vi "ASDA-A2.vi"(5 "Dec":i32, 6 "Address":u16(ring) items=["1", "2"], 7 "Acc":i32, 8 "Torque\\Speed":i32, 9 "Mode":T1(ring)=enum."Set Speed", 10 "VISA resource name":refnum<visa-resource-name>="COM1") -> (1 "Speed":i32, 2 "Error":bool)   [LabVIEW 2024]
panel:
  out "substring":string
  out "crc check result":string
  out "Tact Time":u32
  out "send string":string
  out "Numeric":u8 format="%.0x"
  out "read string":string
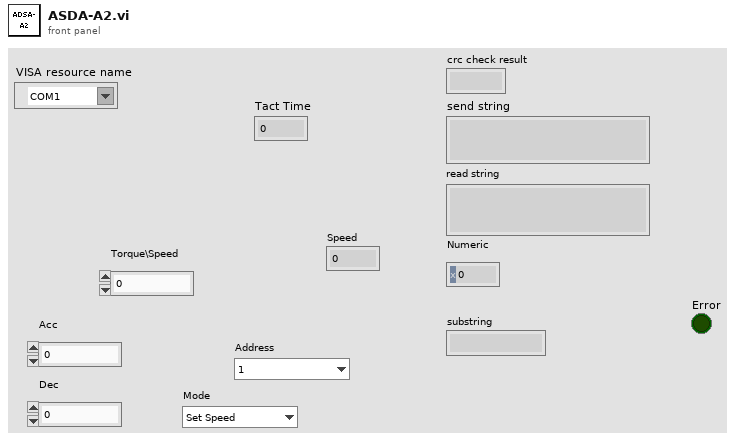
[diagram p1: front panel]
types:
  T1 = enum16{"Set Torque", "Set Speed", "Read Speed", "Set Acc/Dec"}
  T2 = cluster{"VISA resource name":refnum<visa-resource-name>, "baud rate":u32, "data bits":u16, "parity":u16, "stop bits":u16, "flow control":u16, "Read TimeOut (ms)":u32, "Byte Read Count(999Exit)":u32, "Read End Str":bool, "End String":string}
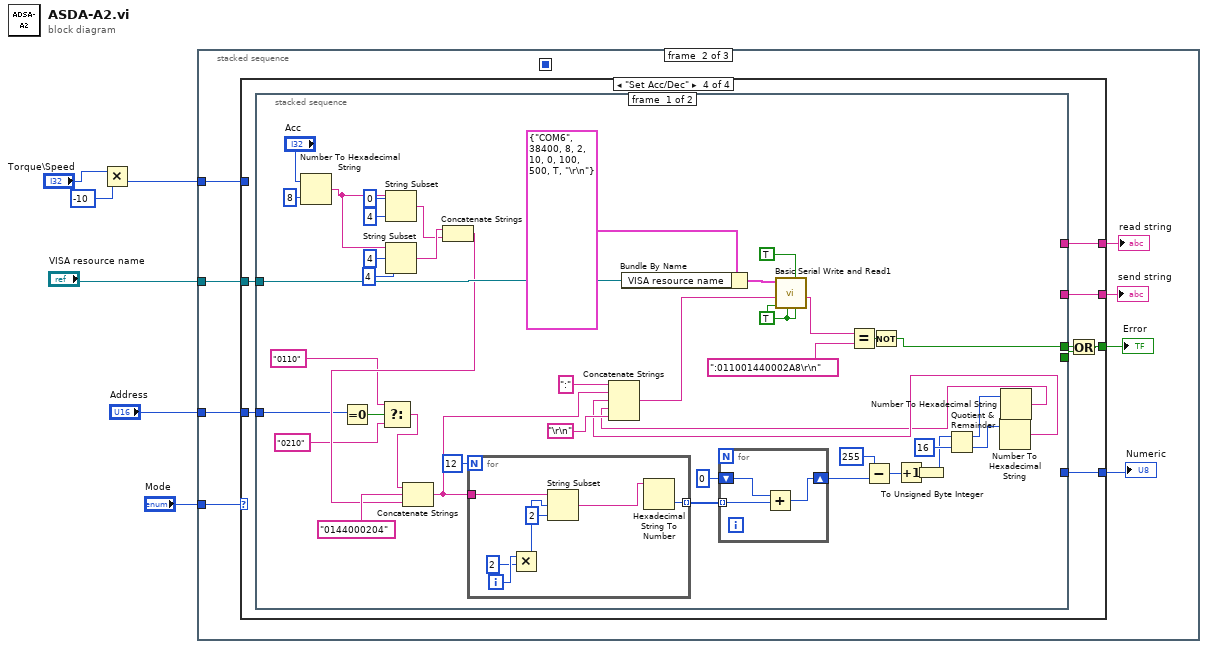
[diagram p0: block diagram]
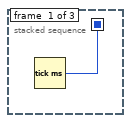
[diagram p2: hidden frame]
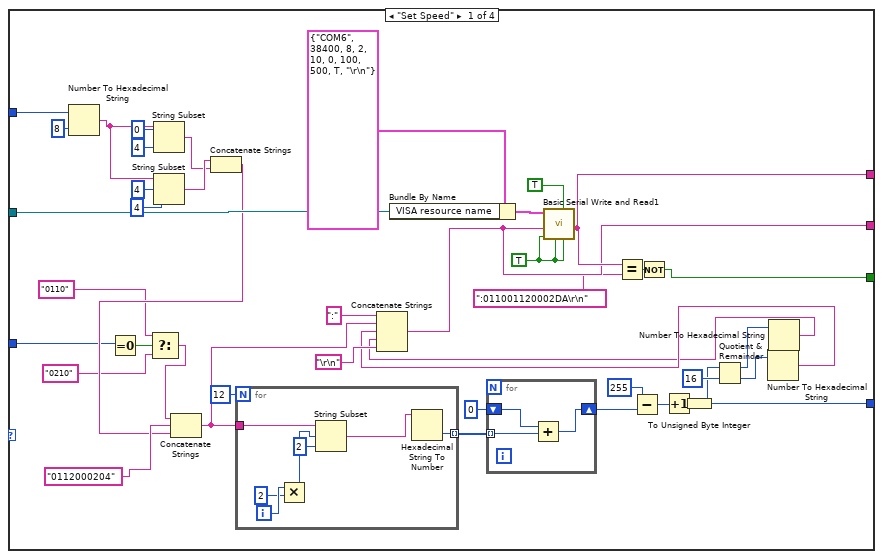
[diagram p3: hidden frame]
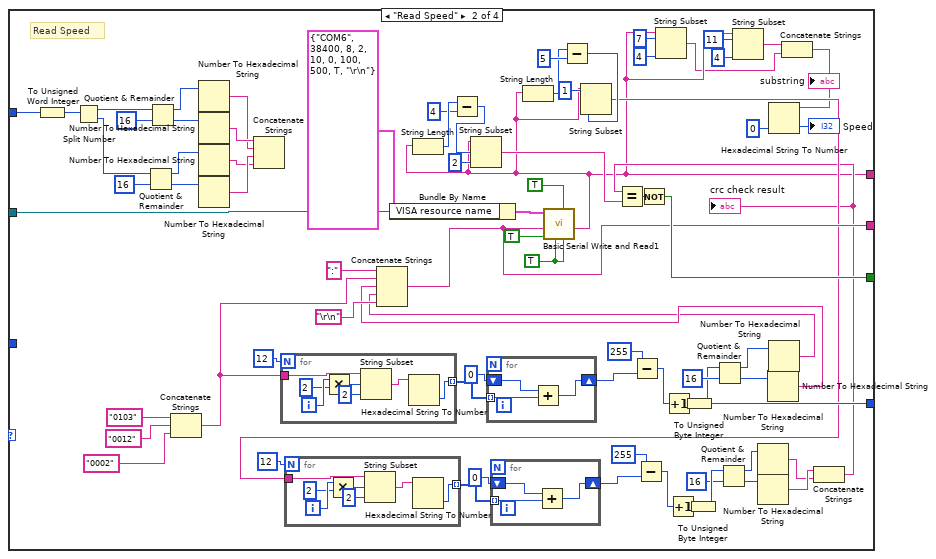
[diagram p4: hidden frame]
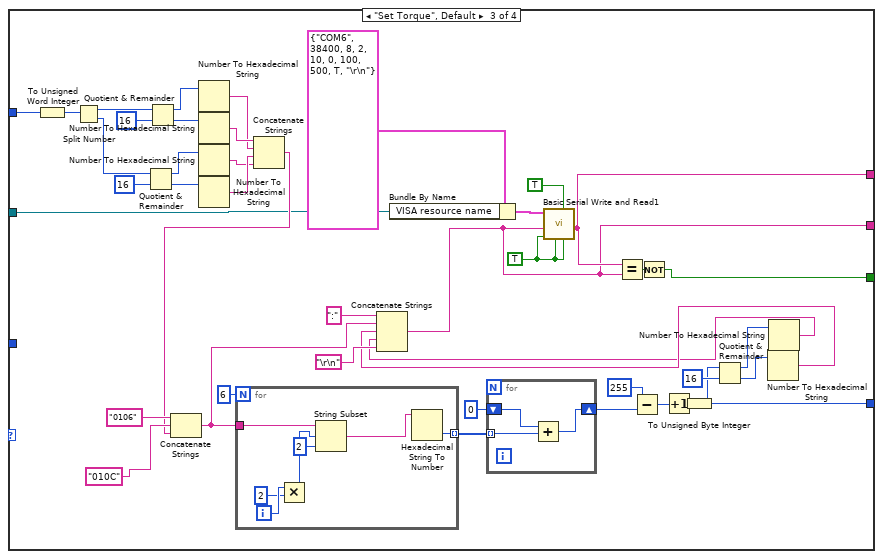
[diagram p5: hidden frame]
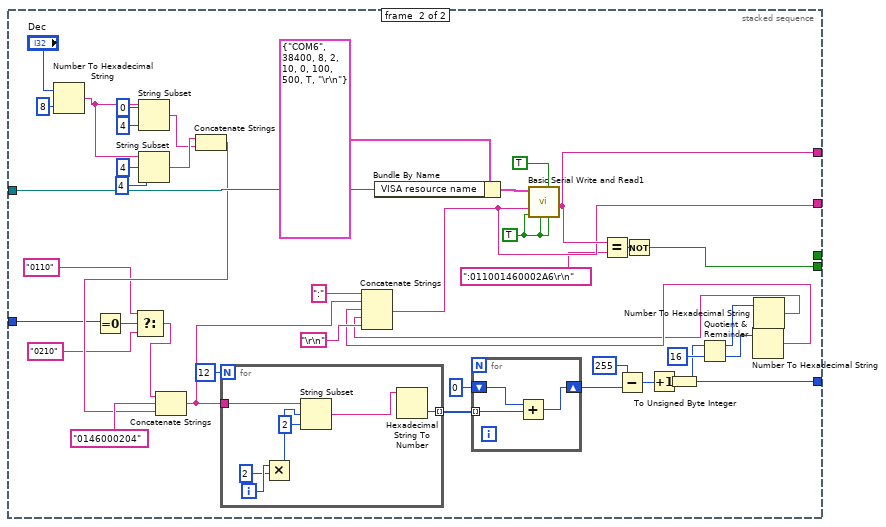
[diagram p6: hidden frame]
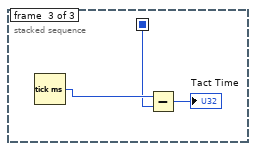
[diagram p7: hidden frame]
diagram:
  n1 = Multiply(x="Torque\\Speed", y=-10) -> (x*y=w3:i32)
  n2 = stacked-sequence {
    seq-local: [w7 _ _] -> [_ _ w329]
    tunnel: w3 -> [_ w15 _]
    tunnel: "VISA resource name" -> [_ w14 _]
    tunnel: "Mode" -> [_ w13 _]
    tunnel: "Address" -> [_ w8 _]
    frame #0 {
      n3 = Tick Count (ms)() -> (millisecond timer value=w7:u32)
    }
    frame #1 {
      n4 = case shown="\"Set Acc/Dec\"" w13 {
        tunnel: w15 -> [w32 w126 w187 _]
        tunnel: w14 -> [w38 w110 w170 w223]
        tunnel: [w36 w108 w168 w222] -> w12
        tunnel: [w35 w107 w167 w218] -> w11
        tunnel: [w34 w73 w166 w221] -> w10
        tunnel: [w33 w106 w165 w220] -> w9
        tunnel: w8 -> [w17 _ _ w219]
        frame "Set Speed" {
          w16 = TRUE ("read")
          n5 = Number To Hexadecimal String(1:i16 8 ("width (-)"), 2:w32) -> (0:w29:string)
          n6 = Equal To 0?(x=w17) -> (x = 0?=w22:bool)
          n7 = Select(t="0110" ("string to write"), s=w22, f="0210" ("string to write")) -> (s? t:f=w20:string)
          n8 = String Subset(string=w29, offset (0)=0, length (rest)=4 ("length (rest)")) -> (substring=w24:string)
          n9 = String Subset(string=w29, offset (0)=4, length (rest)=4 ("length (rest)")) -> (substring=w25:string)
          n10 = Concatenate Strings(w25, w24) -> (w23:string)
          n11 = Concatenate Strings(w20, "0112000204" ("string to write"), w23) -> (w44:string)
          n12 = for {
            N: 12 -> [_]
            tunnel: w44 -> [w64]
            tunnel: [w58] -> w52 mode=indexing
            i -> [w62]
            n13 = Multiply(x=w62, y=2) -> (x*y=w60:i32)
            n14 = String Subset(string=w64, offset (0)=w60, length (rest)=2 ("length (rest)")) -> (substring=w59:string)
            n15 = Hexadecimal String To Number(string=w59) -> (number=w58:u32)  [unwired: 2 in, 1 out]
          }
          n16 = Bundle By Name(cluster=T2 {"VISA resource name"="COM6", "baud rate"=38400, "data bits"=8, "parity"=2, "stop bits"=10, "flow control"=0, "Read TimeOut (ms)"=100, "Byte Read Count(999Exit)"=500, "Read End Str"=TRUE, "End String"="\r\n"} ("Setting"), "VISA resource name"=w38) -> (w39:T2)
          n17 = for {
            shift-right: [w65] -> w49
            shift-left: u32 0 -> [w67]
            tunnel: w52 -> [w66] mode=indexing
            n18 = Add(x=w67, y=w66) -> (x+y=w65:u32)
          }
          n19 = Subtract(x=u32 255, y=w49) -> (x-y=w50:u32)
          n20 = Increment(x=w50) -> (x+1=w48:u32)
          n21 = To Unsigned Byte Integer(number=w48) -> (unsigned 8bit integer=w36:u8)
          n22 = Quotient & Remainder(x=w36, y=u32 16) -> (x-y*floor(x/y)=w46:u32, floor(x/y)=w45:u32)
          n23 = Number To Hexadecimal String(2:w45) -> (0:w42:string)  [unwired: 1 in]
          n24 = Number To Hexadecimal String(2:w46) -> (0:w41:string)  [unwired: 1 in]
          n25 = Concatenate Strings(":" ("string to write"), w44, w42, w41, "\r\n") -> (w33:string)
          n26 = call "Basic Serial Write and Read1.vi"("read"=w16, "write"=TRUE, "Close"=w16, "Open"=w16, "string to write"=w33, "Setting"=w39) -> ("read string"=w34:string)  [unwired: 3 in, 2 out]
          n27 = Equal?(x=w34, y=":011001120002DA\r\n") -> (x = y?=w37:bool)
          n28 = Not(x=w37) -> (.not. x?=w35:bool)
        }
        frame "Read Speed" {
          w68 = TRUE ("read")
          # "Read Speed"
          n29 = To Unsigned Word Integer(number=w126) -> (unsigned 16bit integer=w125:u16)
          n30 = Split Number(x=w125) -> (hi(x)=w122:u8, lo(x)=w117:u8)
          n31 = Quotient & Remainder(x=w117, y=u8 16) -> (x-y*floor(x/y)=w119:u8, floor(x/y)=w118:u8)
          n32 = Quotient & Remainder(x=w122, y=u8 16) -> (x-y*floor(x/y)=w123:u8, floor(x/y)=w124:u8)
          n33 = Concatenate Strings("0103" ("string to write"), "0012" ("string"), "0002" ("string")) -> (w130:string)
          n34 = Number To Hexadecimal String(2:w123) -> (0:w115:string)  [unwired: 1 in]
          n35 = Number To Hexadecimal String(2:w124) -> (0:w116:string)  [unwired: 1 in]
          n36 = Number To Hexadecimal String(2:w119) -> (0:w113:string)  [unwired: 1 in]
          n37 = Number To Hexadecimal String(2:w118) -> (0:w114:string)  [unwired: 1 in]
          n38 = Concatenate Strings(w116, w115, w114, w113) -> ()  [unwired: 1 out]
          n39 = for {
            N: 12 -> [_]
            tunnel: w130 -> [w160]
            tunnel: [w154] -> w138 mode=indexing
            i -> [w158]
            n40 = Multiply(x=w158, y=2) -> (x*y=w156:i32)
            n41 = String Subset(string=w160, offset (0)=w156, length (rest)=2 ("length (rest)")) -> (substring=w155:string)
            n42 = Hexadecimal String To Number(string=w155) -> (number=w154:u32)  [unwired: 2 in, 1 out]
          }
          n43 = Bundle By Name(cluster=T2 {"VISA resource name"="COM6", "baud rate"=38400, "data bits"=8, "parity"=2, "stop bits"=10, "flow control"=0, "Read TimeOut (ms)"=100, "Byte Read Count(999Exit)"=500, "Read End Str"=TRUE, "End String"="\r\n"} ("Setting"), "VISA resource name"=w110) -> (w111:T2)
          n44 = for {
            shift-right: [w161] -> w135
            shift-left: u32 0 -> [w163]
            tunnel: w138 -> [w162] mode=indexing
            n45 = Add(x=w163, y=w162) -> (x+y=w161:u32)
          }
          n46 = Subtract(x=u32 255, y=w135) -> (x-y=w136:u32)
          n47 = Increment(x=w136) -> (x+1=w134:u32)
          n48 = To Unsigned Byte Integer(number=w134) -> (unsigned 8bit integer=w108:u8)
          n49 = Quotient & Remainder(x=w108, y=u32 16) -> (x-y*floor(x/y)=w132:u32, floor(x/y)=w131:u32)
          n50 = Number To Hexadecimal String(2:w131) -> (0:w128:string)  [unwired: 1 in]
          n51 = Number To Hexadecimal String(2:w132) -> (0:w127:string)  [unwired: 1 in]
          n52 = Concatenate Strings(":" ("string to write"), w130, w128, w127, "\r\n") -> (w106:string)
          n53 = call "Basic Serial Write and Read1.vi"("read"=w68, "write"=TRUE, "Close"=w68, "Open"=TRUE, "string to write"=w106, "Setting"=w111) -> ("read string"=w73:string)  [unwired: 3 in, 2 out]
          n54 = String Length(string=w73) -> (length=w102:i32)
          n55 = Subtract(x=w102, y=4) -> (x-y=w100:i32)
          n56 = String Subset(string=w73, offset (0)=w100, length (rest)=2 ("length (rest)")) -> (substring=w81:string)
          n57 = String Length(string=w73) -> (length=w97:i32)
          n58 = Subtract(x=w97, y=5) -> (x-y=w95:i32)
          n59 = String Subset(string=w73, offset (0)=1, length (rest)=w95) -> (substring=w83:string)
          n60 = for {
            N: 12 -> [_]
            tunnel: w83 -> [w150]
            tunnel: [w144] -> w86 mode=indexing
            i -> [w148]
            n61 = Multiply(x=w148, y=2) -> (x*y=w146:i32)
            n62 = String Subset(string=w150, offset (0)=w146, length (rest)=2 ("length (rest)")) -> (substring=w145:string)
            n63 = Hexadecimal String To Number(string=w145) -> (number=w144:u32)  [unwired: 2 in, 1 out]
          }
          n64 = for {
            shift-right: [w151] -> w89
            shift-left: u32 0 -> [w153]
            tunnel: w86 -> [w152] mode=indexing
            n65 = Add(x=w153, y=w152) -> (x+y=w151:u32)
          }
          n66 = Subtract(x=u32 255, y=w89) -> (x-y=w88:u32)
          n67 = String Subset(string=w73, offset (0)=7, length (rest)=4 ("length (rest)")) -> (substring=w71:string)
          n68 = Increment(x=w88) -> (x+1=w90:u32)
          n69 = To Unsigned Byte Integer(number=w90) -> (unsigned 8bit integer=w94:u8)
          n70 = Quotient & Remainder(x=w94, y=u32 16) -> (x-y*floor(x/y)=w92:u32, floor(x/y)=w93:u32)
          n71 = String Subset(string=w73, offset (0)=11, length (rest)=4 ("length (rest)")) -> (substring=w72:string)
          n72 = Number To Hexadecimal String(2:w92) -> (0:w79:string)  [unwired: 1 in]
          n73 = Number To Hexadecimal String(2:w93) -> (0:w80:string)  [unwired: 1 in]
          n74 = Concatenate Strings(w72, w71) -> (w70:string)
          "substring" <- w70
          n75 = Hexadecimal String To Number(string=w70, default (0uL)=0 ("default (0 U32)")) -> (number=→"Speed":i32)  [unwired: 1 in, 1 out]
          n76 = Concatenate Strings(w80, w79) -> (w82:string)
          "crc check result" <- w82
          n77 = Equal?(x=w82, y=w81) -> (x = y?=w109:bool)
          n78 = Not(x=w109) -> (.not. x?=w107:bool)
        }
        frame "Set Torque", Default {
          w164 = TRUE ("read")
          n79 = To Unsigned Word Integer(number=w187) -> (unsigned 16bit integer=w186:u16)
          n80 = Split Number(x=w186) -> (hi(x)=w183:u8, lo(x)=w178:u8)
          n81 = Quotient & Remainder(x=w178, y=u8 16) -> (x-y*floor(x/y)=w180:u8, floor(x/y)=w179:u8)
          n82 = Quotient & Remainder(x=w183, y=u8 16) -> (x-y*floor(x/y)=w184:u8, floor(x/y)=w185:u8)
          n83 = Number To Hexadecimal String(2:w184) -> (0:w176:string)  [unwired: 1 in]
          n84 = Number To Hexadecimal String(2:w185) -> (0:w177:string)  [unwired: 1 in]
          n85 = Number To Hexadecimal String(2:w180) -> (0:w174:string)  [unwired: 1 in]
          n86 = Number To Hexadecimal String(2:w179) -> (0:w175:string)  [unwired: 1 in]
          n87 = Concatenate Strings(w177, w176, w175, w174) -> (w173:string)
          n88 = Concatenate Strings("0106" ("string to write"), "010C" ("string to write"), w173) -> (w191:string)
          n89 = for {
            N: 6 -> [_]
            tunnel: w191 -> [w212]
            tunnel: [w206] -> w199 mode=indexing
            i -> [w210]
            n90 = Multiply(x=w210, y=2) -> (x*y=w208:i32)
            n91 = String Subset(string=w212, offset (0)=w208, length (rest)=2 ("length (rest)")) -> (substring=w207:string)
            n92 = Hexadecimal String To Number(string=w207) -> (number=w206:u32)  [unwired: 2 in, 1 out]
          }
          n93 = Bundle By Name(cluster=T2 {"VISA resource name"="COM6", "baud rate"=38400, "data bits"=8, "parity"=2, "stop bits"=10, "flow control"=0, "Read TimeOut (ms)"=100, "Byte Read Count(999Exit)"=500, "Read End Str"=TRUE, "End String"="\r\n"} ("Setting"), "VISA resource name"=w170) -> (w171:T2)
          n94 = for {
            shift-right: [w213] -> w196
            shift-left: u8 0 -> [w215]
            tunnel: w199 -> [w214] mode=indexing
            n95 = Add(x=w215, y=w214) -> (x+y=w213:u32)
          }
          n96 = Subtract(x=255, y=w196) -> (x-y=w197:u32)
          n97 = Increment(x=w197) -> (x+1=w195:u32)
          n98 = To Unsigned Byte Integer(number=w195) -> (unsigned 8bit integer=w168:u8)
          n99 = Quotient & Remainder(x=w168, y=u32 16) -> (x-y*floor(x/y)=w193:u32, floor(x/y)=w192:u32)
          n100 = Number To Hexadecimal String(2:w192) -> (0:w189:string)  [unwired: 1 in]
          n101 = Number To Hexadecimal String(2:w193) -> (0:w188:string)  [unwired: 1 in]
          n102 = Concatenate Strings(":" ("string to write"), w191, w189, w188, "\r\n") -> (w165:string)
          n103 = call "Basic Serial Write and Read1.vi"("read"=w164, "write"=TRUE, "Close"=w164, "Open"=w164, "string to write"=w165, "Setting"=w171) -> ("read string"=w166:string)  [unwired: 3 in, 2 out]
          n104 = Equal?(x=w166, y=w165) -> (x = y?=w169:bool)
          n105 = Not(x=w169) -> (.not. x?=w167:bool)
        }
        frame "Set Acc/Dec" {
          n106 = stacked-sequence {
            tunnel: w223 -> [w246 w298]
            tunnel: [_ w296] -> w222
            tunnel: [w243 _] -> w217
            tunnel: [_ w295] -> w221
            tunnel: [_ w294] -> w220
            tunnel: w219 -> [w225 w279]
            tunnel: [_ w277] -> w216
            frame #0 {
              w224 = TRUE ("read")
              n107 = Number To Hexadecimal String(1:i16 8 ("width (-)"), 2:"Acc") -> (0:w238:string)
              n108 = Equal To 0?(x=w225) -> (x = 0?=w231:bool)
              n109 = Select(t="0110" ("string to write"), s=w231, f="0210" ("string to write")) -> (s? t:f=w229:string)
              n110 = String Subset(string=w238, offset (0)=0, length (rest)=4 ("length (rest)")) -> (substring=w233:string)
              n111 = String Subset(string=w238, offset (0)=4, length (rest)=4 ("length (rest)")) -> (substring=w234:string)
              n112 = Concatenate Strings(w234, w233) -> (w232:string)
              n113 = Concatenate Strings(w229, "0144000204" ("string to write"), w232) -> (w252:string)
              n114 = for {
                N: 12 -> [_]
                tunnel: w252 -> [w272]
                tunnel: [w266] -> w260 mode=indexing
                i -> [w270]
                n115 = Multiply(x=w270, y=2) -> (x*y=w268:i32)
                n116 = String Subset(string=w272, offset (0)=w268, length (rest)=2 ("length (rest)")) -> (substring=w267:string)
                n117 = Hexadecimal String To Number(string=w267) -> (number=w266:u32)  [unwired: 2 in, 1 out]
              }
              n118 = Bundle By Name(cluster=T2 {"VISA resource name"="COM6", "baud rate"=38400, "data bits"=8, "parity"=2, "stop bits"=10, "flow control"=0, "Read TimeOut (ms)"=100, "Byte Read Count(999Exit)"=500, "Read End Str"=TRUE, "End String"="\r\n"} ("Setting"), "VISA resource name"=w246) -> (w247:T2)
              n119 = for {
                shift-right: [w273] -> w257
                shift-left: u32 0 -> [w275]
                tunnel: w260 -> [w274] mode=indexing
                n120 = Add(x=w275, y=w274) -> (x+y=w273:u32)
              }
              n121 = Subtract(x=u32 255, y=w257) -> (x-y=w258:u32)
              n122 = Increment(x=w258) -> (x+1=w256:u32)
              n123 = To Unsigned Byte Integer(number=w256) -> (unsigned 8bit integer=w244:u8)
              n124 = Quotient & Remainder(x=w244, y=u32 16) -> (x-y*floor(x/y)=w254:u32, floor(x/y)=w253:u32)
              n125 = Number To Hexadecimal String(2:w253) -> (0:w250:string)  [unwired: 1 in]
              n126 = Number To Hexadecimal String(2:w254) -> (0:w249:string)  [unwired: 1 in]
              n127 = Concatenate Strings(":" ("string to write"), w252, w250, w249, "\r\n") -> (w241:string)
              n128 = call "Basic Serial Write and Read1.vi"("read"=w224, "write"=TRUE, "Close"=w224, "Open"=w224, "string to write"=w241, "Setting"=w247) -> ("read string"=w242:string)  [unwired: 3 in, 2 out]
              n129 = Equal?(x=w242, y=":011001440002A8\r\n") -> (x = y?=w245:bool)
              n130 = Not(x=w245) -> (.not. x?=w243:bool)
            }
            frame #1 {
              w276 = TRUE ("read")
              n131 = Number To Hexadecimal String(1:i16 8 ("width (-)"), 2:"Dec") -> (0:w291:string)
              n132 = Equal To 0?(x=w279) -> (x = 0?=w284:bool)
              n133 = Select(t="0110" ("string to write"), s=w284, f="0210" ("string to write")) -> (s? t:f=w282:string)
              n134 = String Subset(string=w291, offset (0)=0, length (rest)=4 ("length (rest)")) -> (substring=w286:string)
              n135 = String Subset(string=w291, offset (0)=4, length (rest)=4 ("length (rest)")) -> (substring=w287:string)
              n136 = Concatenate Strings(w287, w286) -> (w285:string)
              n137 = Concatenate Strings(w282, "0146000204" ("string to write"), w285) -> (w304:string)
              n138 = for {
                N: 12 -> [_]
                tunnel: w304 -> [w324]
                tunnel: [w318] -> w312 mode=indexing
                i -> [w322]
                n139 = Multiply(x=w322, y=2) -> (x*y=w320:i32)
                n140 = String Subset(string=w324, offset (0)=w320, length (rest)=2 ("length (rest)")) -> (substring=w319:string)
                n141 = Hexadecimal String To Number(string=w319) -> (number=w318:u32)  [unwired: 2 in, 1 out]
              }
              n142 = Bundle By Name(cluster=T2 {"VISA resource name"="COM6", "baud rate"=38400, "data bits"=8, "parity"=2, "stop bits"=10, "flow control"=0, "Read TimeOut (ms)"=100, "Byte Read Count(999Exit)"=500, "Read End Str"=TRUE, "End String"="\r\n"} ("Setting"), "VISA resource name"=w298) -> (w299:T2)
              n143 = for {
                shift-right: [w325] -> w309
                shift-left: u32 0 -> [w327]
                tunnel: w312 -> [w326] mode=indexing
                n144 = Add(x=w327, y=w326) -> (x+y=w325:u32)
              }
              n145 = Subtract(x=u32 255, y=w309) -> (x-y=w310:u32)
              n146 = Increment(x=w310) -> (x+1=w308:u32)
              n147 = To Unsigned Byte Integer(number=w308) -> (unsigned 8bit integer=w296:u8)
              n148 = Quotient & Remainder(x=w296, y=u32 16) -> (x-y*floor(x/y)=w306:u32, floor(x/y)=w305:u32)
              n149 = Number To Hexadecimal String(2:w305) -> (0:w302:string)  [unwired: 1 in]
              n150 = Number To Hexadecimal String(2:w306) -> (0:w301:string)  [unwired: 1 in]
              n151 = Concatenate Strings(":" ("string to write"), w304, w302, w301, "\r\n") -> (w294:string)
              n152 = call "Basic Serial Write and Read1.vi"("read"=w276, "write"=TRUE, "Close"=w276, "Open"=w276, "string to write"=w294, "Setting"=w299) -> ("read string"=w295:string)  [unwired: 3 in, 2 out]
              n153 = Equal?(x=w295, y=":011001460002A6\r\n") -> (x = y?=w297:bool)
              n154 = Not(x=w297) -> (.not. x?=w277:bool)
            }
          }
          n155 = Or(x=w217, y=w216) -> (x .or. y?=w218:bool)
        }
      }
      "Numeric" <- w12
      "Error" <- w11
      "read string" <- w10
      "send string" <- w9
    }
    frame #2 {
      n156 = Tick Count (ms)() -> (millisecond timer value=w330:u32)
      n157 = Subtract(x=w330, y=w329) -> (x-y=→"Tact Time":u32)
    }
  }
